vi "Write Auto LED Control.vi"(8 "error in (no error)":errorcluster, 10 "Auto LED Control":bool, 11 "LINX-AutomationHat in":refnum<class "LINX-AutomationHat.lvclass">) -> (0 "error out":errorcluster, 3 "LINX-AutomationHat out":refnum<class "LINX-AutomationHat.lvclass">)   [LabVIEW 2020, in "LINX-AutomationHat.lvclass"]
uses:
  LINX-AutomationHat.lvclass
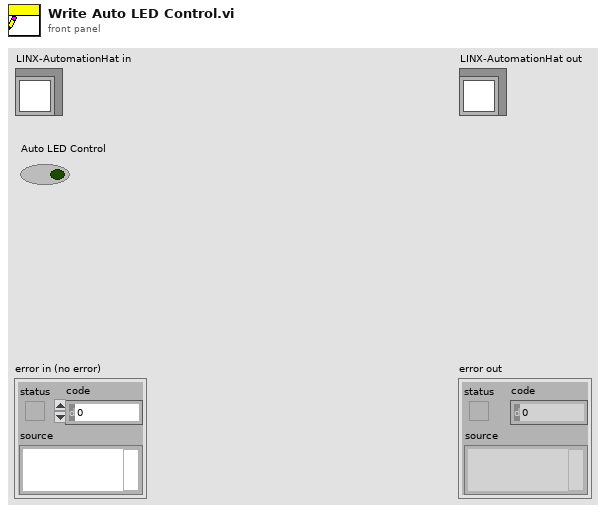
[diagram p1: front panel]
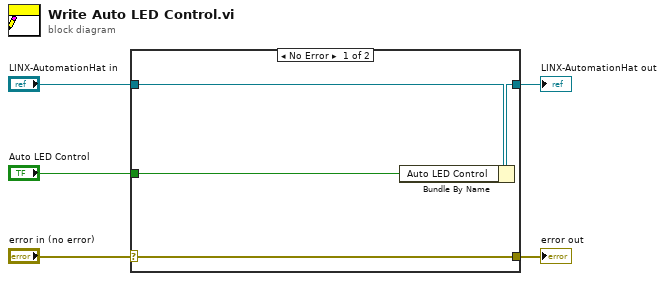
[diagram p0: block diagram]
diagram:
  n1 = case shown="No Error" "error in (no error)" {
    selector: "error in (no error)" -> [w9 w10]
    tunnel: [w9 w10] -> w4
    tunnel: [w7 w11] -> w2
    tunnel: "LINX-AutomationHat in" -> [w8 w11]
    tunnel: "Auto LED Control" -> [w6 _]
    frame No Error {
      n2 = Bundle By Name(cluster=w8, "Auto LED Control"=w6) -> (w7:refnum<class "LINX-AutomationHat.lvclass">)
    }
    frame Error {
    }
  }
  "error out" <- w4
  "LINX-AutomationHat out" <- w2
